vi "Paint_Center_of_Particle-7.vi"(0 "[IN] Initialized Image":T4, 1 "[IN] AVI Refnum":T3, 3 "[IN] Image Type":T2 items=["Grayscale (U8)", "Grayscale (I16)", "Grayscale (SGL)", "Complex (CSG)", "RGB (U32)", "HSL (U32)", "RGB (U64)", "Grayscale (U16)"], 5 "[IN] Frame Number":u32, 9 "[IN] Array of X,Y":dbl[](array[numeric]), 11 "error IN":errorcluster, 12 "[IN] Filtering Settings":T1, 13 "Keep Nega-\ntive Values?":bool, 14 "[IN] # Channel":u8) -> (4 "[OUT] Image Dst":T4, 15 "error OUT":errorcluster)   [LabVIEW 2013]
doc: "SubVI make a picture of all localized particles in a frame"
uses:
  <vilib>/vision/Image Controls.llb/IMAQ Image.ctl
  <vilib>/vision/Avi.llb/IMAQ AVI2 Refnum.ctl
  <vilib>/vision/NI_Vision_Development_Module.lvlib
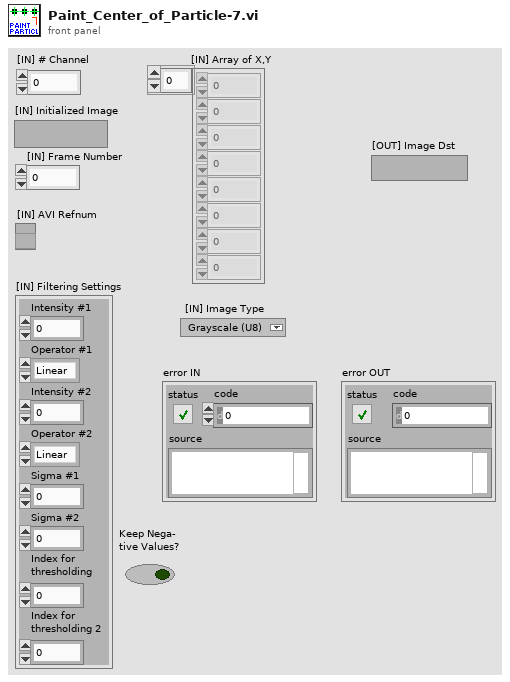
[diagram p1: front panel]
types:
  T1 = cluster{"Intensity #1":sgl, "Operator #1":enum32{"Linear", "Log", "Exp", "Square", "Square root", "Power X", "Power 1/X"}, "Intensity #2":sgl, "Operator #2":enum32{"Linear", "Log", "Exp", "Square", "Square root", "Power X", "Power 1/X"}, "Sigma #1":dbl, "Sigma #2":dbl, "Index for \nthresholding":u8, "Index for \nthresholding 2":u8}
  T2 = typedef "Image Type" = u32
  T3 = typedef "IMAQ AVI2 Refnum.ctl" = refnum<k20>
  T4 = typedef "IMAQ Image.ctl" = refnum<image>
  T5 = enum32{"Linear", "Log", "Exp", "Square", "Square root", "Power X", "Power 1/X"}
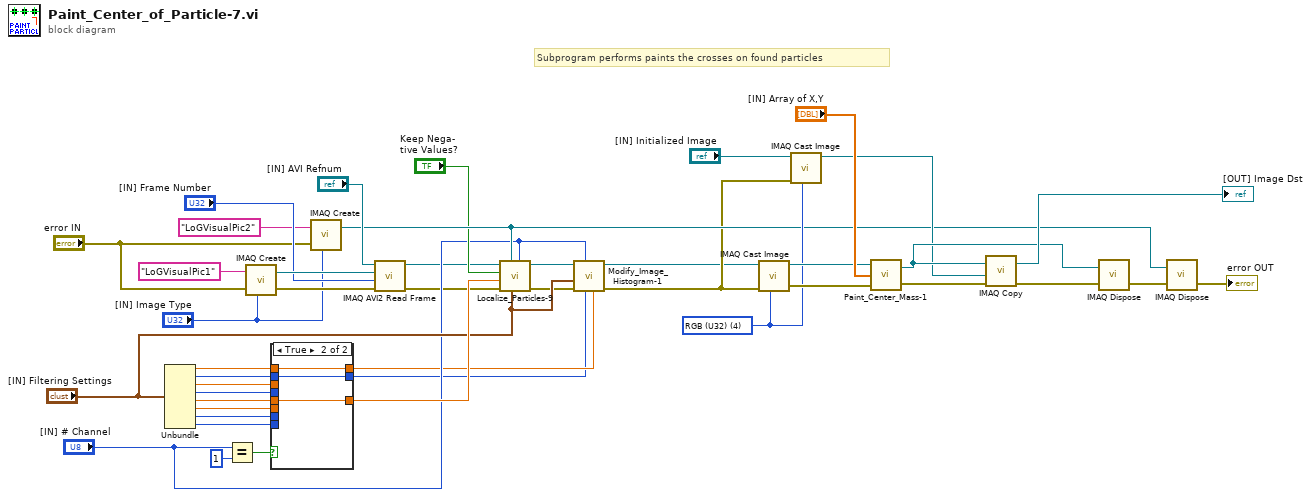
[diagram p0: block diagram]
diagram:
  w18 = T2 4 items=["Grayscale (U8)", "Grayscale (I16)", "Grayscale (SGL)", "Complex (CSG)", "RGB (U32)", "HSL (U32)", "RGB (U64)", "Grayscale (U16)"] ("Image Type")
  # "Subprogram performs paints the crosses on found particles"
  n1 = Unbundle("[IN] Filtering Settings") -> ("Intensity #1"=w38:sgl, "Operator #1"=w39:T5, "Intensity #2"=w40:sgl, "Operator #2"=w41:T5, "Sigma #1"=w25:dbl, "Sigma #2"=w24:dbl, "Index for \nthresholding"=w23:u8, "Index for \nthresholding 2"=w22:u8)
  n2 = Equal?(x="[IN] # Channel", y=u8 1) -> (x = y?=w42:bool)
  n3 = call "IMAQ Create"("Image Name"="LoGVisualPic1", "Image Type"="[IN] Image Type", "error in (no error)"="error IN") -> ("New Image"=w35:T4, "error out"=w34:errorcluster)  [unwired: 2 in]
  n4 = case shown="True" w42 {
    tunnel: w41 -> [w45 _]
    tunnel: w40 -> [w46 _]
    tunnel: w39 -> [_ w48]
    tunnel: w38 -> [_ w49]
    tunnel: [w46 w49] -> w6
    tunnel: [w45 w48] -> w5
    tunnel: w25 -> [_ w47]
    tunnel: w24 -> [w44 _]
    tunnel: [w44 w47] -> w12
    tunnel: w23 -> [_ _]
    tunnel: w22 -> [_ _]
    frame False {
    }
    frame True {
    }
  }
  n5 = call "IMAQ Create"("Image Name"="LoGVisualPic2", "Image Type"="[IN] Image Type", "error in (no error)"="error IN") -> ("New Image"=w13:T4)  [unwired: 2 in, 1 out]
  n6 = call "IMAQ AVI2 Read Frame"("error in (no error)"=w34, "Frame Number"="[IN] Frame Number", "Image"=w35, "AVI Refnum"="[IN] AVI Refnum") -> ("error out"=w4:errorcluster, "Image Out"=w3:T4)  [unwired: 5 in, 1 out]
  n7 = call "Localize_Particles-9.vi"("# channel"="[IN] # Channel", "[IN] Filtering Settings"="[IN] Filtering Settings", "[IN] Destination Image"=w13, "error IN"=w4, "[IN] Sigma"=w12, "Keep Nega-\ntive Values?"="Keep Nega-\ntive Values?", "[IN] Frame"=w3) -> ("error OUT"=w8:errorcluster, "[OUT] LoG Processed Image"=w10:T4)  [unwired: 1 in, 1 out]
  n8 = call "Modify_Image_Histogram-1.vi"("[IN] Parameter"=w6, "[IN] Operator"=w5, "# channel"="[IN] # Channel", "error IN"=w8, "[IN] Filtering Settings"="[IN] Filtering Settings", "[IN] LoG Processed Image"=w10) -> ("error OUT"=w2:errorcluster, "[OUT] Histogram Modified Image"=w1:T4)  [unwired: 2 in, 2 out]
  n9 = call "IMAQ Cast Image"("Image Type"=w18, "error in (no error)"=w2, "Image Src"=w1) -> ("error out"=w20:errorcluster, "Image Dst Out"=w21:T4)  [unwired: 7 in]
  n10 = call "IMAQ Cast Image"("Image Type"=w18, "error in (no error)"=w2, "Image Src"="[IN] Initialized Image") -> ("Image Dst Out"=w17:T4)  [unwired: 7 in, 1 out]
  n11 = call "Paint_Center_Mass-1.vi"("error IN"=w20, "Array of Points IN"="[IN] Array of X,Y", "Image IN"=w21) -> ("error OUT"=w30:errorcluster, "Image OUT"=w29:T4)
  n12 = call "IMAQ Copy"("error in (no error)"=w30, "Image Dst"=w17, "Image Src"=w29) -> ("error out"=w33:errorcluster, "Image Dst Out"=→"[OUT] Image Dst":T4)  [unwired: 3 in]
  n13 = call "IMAQ Dispose"("Image"=w29, "error in (no error)"=w33) -> ("error out"=w16:errorcluster)  [unwired: 4 in]
  n14 = call "IMAQ Dispose"("Image"=w13, "error in (no error)"=w16) -> ("error out"=→"error OUT":errorcluster)  [unwired: 4 in]
